vi "Get Alias-Free Connection Endpoint.vi"(9 "type":enum16{"Source", "Destination", "Neither"}(ring), 10 "Connection row":T1, 11 "Channel Editor State":T2={"Modules and Connections"=[{" Module Path"="", "Short Module Path"="", "Product Name"="", "Possible Connections"=[], "Missing"=FALSE}, {" Module Path"="", "Short Module Path"="", "Product Name"="", "Possible Connections"=[], "Missing"=FALSE}], "Alias Mappings UI"=[], "Mappings by Module UI"=[]}) -> (3 "Endpoint (Model) String":string)   [LabVIEW 2020, in "Routing and Faulting System Explorer.lvlib"]
uses:
  Routing and Faulting System Explorer.lvlib
  Channel Editor State.ctl
  Possible Connections.ctl
  Shared/Routing and Faulting Hardware API/Types/Possible Connections for Endpoint.ctl
  Shared/Alias Mapping.ctl
  Shared/Alias Endpoint.ctl
  Alias Map by Module.ctl
  Connection Row.ctl
  Shared/Routing and Faulting Shared.lvlib
  Shared/Routing and Faulting Hardware API/Routing and Faulting Hardware API.lvlib
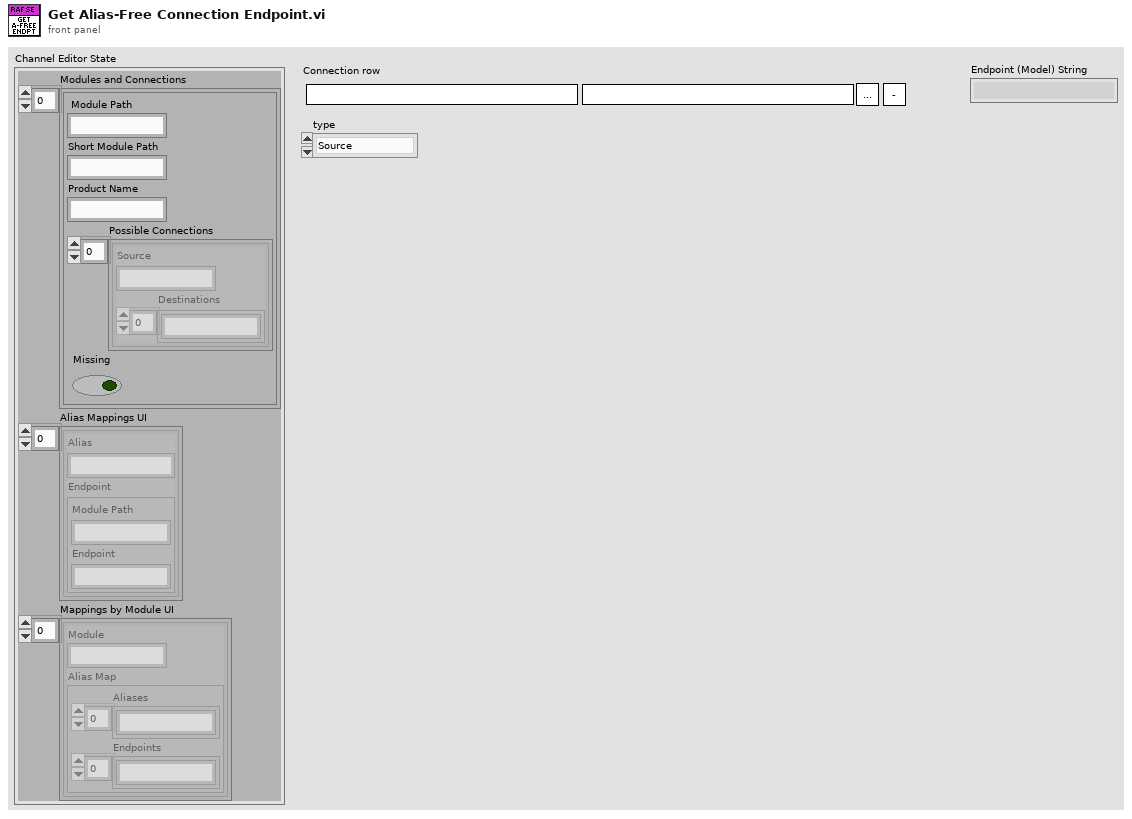
[diagram p1: front panel]
types:
  T1 = typedef "Routing and Faulting System Explorer.lvlib/Connection Row.ctl" = cluster{"Source":string, "Destination":string, "Edit":bool, "Remove":bool}
  T2 = typedef "Routing and Faulting System Explorer.lvlib/Channel Editor State.ctl" = cluster{"Modules and Connections":T3[], "Alias Mappings UI":T5[], "Mappings by Module UI":T7[]}
  T3 = typedef "Routing and Faulting System Explorer.lvlib/Possible Connections.ctl" = cluster{" Module Path":string, "Short Module Path":string, "Product Name":string, "Possible Connections":T4[], "Missing":bool}
  T4 = typedef "Routing and Faulting Hardware API.lvlib/Possible Connections for Endpoint.ctl" = cluster{"Source":string, "Destinations":string[]}
  T5 = typedef "Routing and Faulting Shared.lvlib/Alias Mapping.ctl" = cluster{"Alias":string, "Endpoint":T6}
  T6 = typedef "Routing and Faulting Shared.lvlib/Alias Endpoint.ctl" = cluster{"Module Path":string, "Endpoint":string}
  T7 = typedef "Routing and Faulting System Explorer.lvlib/Alias Map by Module.ctl" = cluster{"Module":string, "Alias Map":cluster{"Aliases":string[], "Endpoints":string[]}}
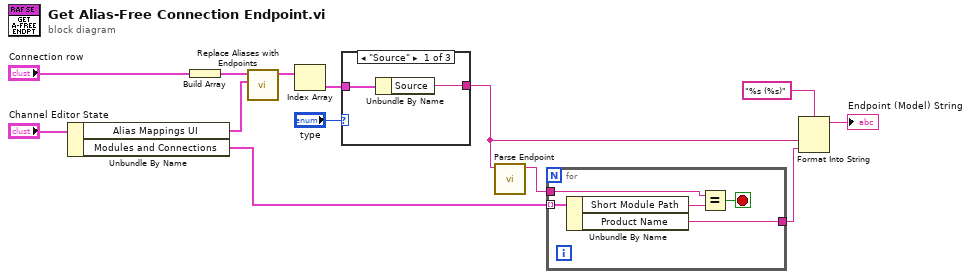
[diagram p0: block diagram]
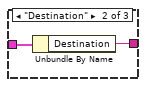
[diagram p2: hidden frame]
diagram:
  n1 = Unbundle By Name("Channel Editor State") -> ("Alias Mappings UI"=w7:T5[], "Modules and Connections"=w6:T3[])
  n2 = Build Array("Connection row") -> (w10:T1[])
  n3 = call "Replace Aliases with Endpoints.vi"("Alias Mappings"=w7, "UI Connections List in"=w10) -> ("UI Connections List out"=w11:T1[])  [unwired: 9 in]
  n4 = Index Array(array=w11) -> (element=w12:T1)  [unwired: 1 in]
  n5 = case shown="\"Source\"" "type" {
    tunnel: w12 -> [w15 w17 _]
    tunnel: [w14 w16 _] -> w3
    frame "Source" {
      n6 = Unbundle By Name(w15) -> ("Source"=w14:string)
    }
    frame "Destination" {
      n7 = Unbundle By Name(w17) -> ("Destination"=w16:string)
    }
    frame "Neither", Default {
    }
  }
  n8 = call "Parse Endpoint.vi"("Module/Endpoint"=w3) -> ("Module"=w5:string)  [unwired: 9 in, 1 out]
  n9 = for {
    tunnel: w6 -> [w22] mode=indexing
    tunnel: w5 -> [w20]
    tunnel: [w18] -> w2
    stop <- w19 stop-if-true
    n10 = Unbundle By Name(w22) -> ("Short Module Path"=w21:string, "Product Name"=w18:string)
    n11 = Equal?(x=w20, y=w21) -> (x = y?=w19:bool)
  }
  n12 = Format Into String(format string="%s (%s)", w3, w2) -> (resulting string=→"Endpoint (Model) String":string)  [unwired: 2 in, 1 out]
